vi "Dynamic call-AOL Z cal wizard.vi"(8 "error in (no error)":errorcluster) -> (0 "error out":errorcluster)   [LabVIEW 2017]
uses:
  Configuration code/Calibration/Globals/gl_Calibration globals.vi
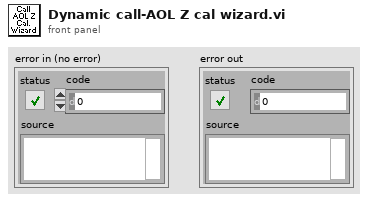
[diagram p1: front panel]
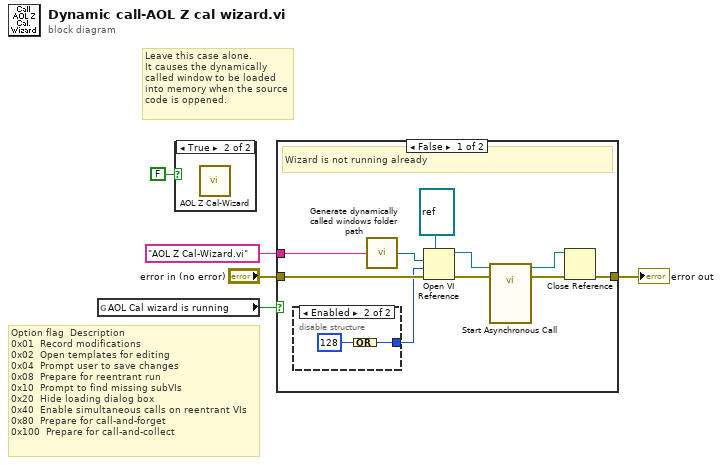
[diagram p0: block diagram]
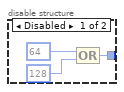
[diagram p3: hidden frame]
diagram:
  # "Leave this case alone.\nIt causes the dynamically called window to be loaded into memory when the source code is oppened."
  # "Option flag \tDescription\n0x01 \tRecord modifications\n0x02 \tOpen templates for editing\n0x04 \tPrompt user to save changes\n0x08 \tPrepare for reentrant run\n0x10 \tPrompt to find missing subVIs\n0x20 \tHide loading dialog box\n0x40 \tEnable simultaneous calls on reentrant VIs\n0x80 \tPrepare for call-and-forget\n0x100 \tPrepare for call-and-collect"
  n1 = global read "gl_Calibration globals.vi" "AOL Cal wizard is running"() -> (w2:bool)
  n2 = case shown="True" FALSE {
    frame False {
    }
    frame True {
      n3 = call "AOL Z Cal-Wizard.vi"() -> ()  [unwired: 12 in]
    }
  }
  n4 = case shown="False" w2 {
    tunnel: "error in (no error)" -> [w15 w21]
    tunnel: [w14 w21] -> w5
    tunnel: "AOL Z Cal-Wizard.vi" ("Error Source") -> [w12 _]
    frame False {
      # "Wizard is not running already"
      n5 = disable-structure shown="Enabled" {
        disable-tunnel: [w18 w20] -> w9
        frame Disabled {
          n6 = Compound Arithmetic op=OR(64, 128) -> (w18:i32)
        }
        frame Enabled {
          n7 = Compound Arithmetic op=OR(128) -> (w20:i32)
        }
      }
      n8 = call "Generate dynamically called windows folder path.vi"("name of dynamically called VI"=w12) -> ("Dynamically called VI path"=w13:path)
      n9 = Open VI Reference(type specifier VI Refnum (for type only)=refnum<vi> refnum, vi path=w13, options=w9, error in (no error)=w15) -> (vi reference=w10:refnum<vi>, error out=w11:errorcluster)  [unwired: 2 in]
      n10 = call-by-ref "Start Asynchronous Call"(reference=w10, error in=w11) -> (reference out=w6:refnum<vi>, error out=w7:errorcluster)  [unwired: 12 in]
      n11 = Close Reference(reference=w6, error in (no error)=w7) -> (error out=w14:errorcluster)
    }
    frame True {
      # "Wizard is already running"
    }
  }
  "error out" <- w5
